vi "Resampler (2 Channel).vi"(5 "CalibrationTable Length-1":u16=799, 7 "ResampleVectorInfo":refnum<k21>="Interpolation Vector Table", 8 "DataValid":bool=TRUE, 11 "Input Data":T2[](array[typedef])=[0.0, 0.0]) -> (0 "Data Valid":bool[](array[boolean]), 3 "Interpolated Data":T1[](array[typedef]))   [LabVIEW 2011]
doc: "This VI resamples input stream to rquired input length of FFT.\n\nTable Length-1 is the length of calibration table. \nIf Input record length is 1600 and processing is done per 2 samples. Then Table-1 = 1600/2-1 = 799"
uses:
  <userlib>/FPGA Library/Code Development/Signal Processing/Interpolation Block/Controls/Interpolation Input Data.ctl
  <userlib>/FPGA Library/Code Development/Signal Processing/Interpolation Block/Controls/Interpolation Output Data.ctl
  <vilib>/rvi/DataTransferAndStorage/Container/Common/niFpgaContainerExecOnDevCompGetState.vi
  <vilib>/rvi/Memory/Memory_Emulation/niFpgaMemoryEmulationValidateCache.vi
  <vilib>/rvi/DataTransferAndStorage/Container/Common/niFpgaContainerGetUniqueNameForEmu.vi
  <vilib>/rvi/Memory/Memory_Emulation/nirvimemoryEmulationManagerCache_InsertValue.vi
  <vilib>/Utility/error.llb/Clear Errors.vi
  <vilib>/rvi/Memory/Memory_Emulation/nirvimemoryEmulationManagerCache_GetValue.vi
  <vilib>/rvi/FXPMathLib/basic elements/FxpDiscreteDelay/XNode/nifxpmath_DiscreteDelay.xnode
  <vilib>/rvi/DataTransferAndStorage/Container/XNode/niFpgaContainer.xnode
  <vilib>/rvi/Memory/Memory_Emulation/niFpgaMemoryEmulationRefIn.vi
  <userlib>/FPGA Library/Code Development/Signal Processing/Interpolation Block/Controls/ResampleVectorInfo (Single Point).ctl
  <userlib>/FPGA Library/Code Development/Signal Processing/Interpolation Block/Controls/ResampleVectorInfo (Multiple Point).ctl
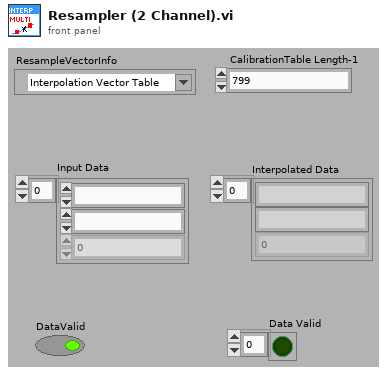
[diagram p1: front panel]
types:
  T1 = typedef "Interpolation Output Data.ctl" = fxp<+/-,19,1>
  T2 = typedef "Interpolation Input Data.ctl" = fxp<+/-,18,1>
  T3 = typedef "ResampleVectorInfo (Multiple Point).ctl" = cluster{"x[n].ResampleInfo":T4, "x[n-1].ResampleInfo":T4}
  T4 = typedef "ResampleVectorInfo (Single Point).ctl" = cluster{"Calc Resample?":bool, "Lambda":fxp<+/-,18,1>}
  T5 = cluster{"x[n].ResampleInfo":cluster{"Calc Resample?":bool, "Lambda":fxp<+/-,18,1>}, "x[n-1].ResampleInfo":cluster{"Calc Resample?":bool, "Lambda":fxp<+/-,18,1>}}
  T6 = cluster{"Calc Resample?":bool, "Lambda":fxp<+/-,18,1>}
  T7 = cluster{"Interpolated Value":T1, "Output Valid":bool}
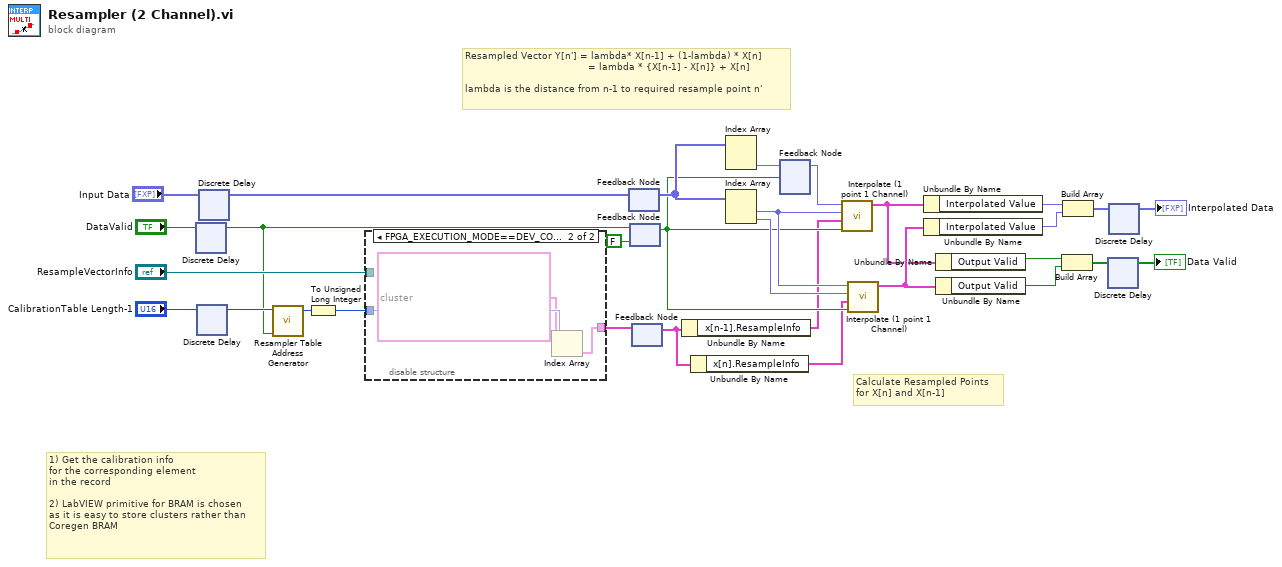
[diagram p0: block diagram]
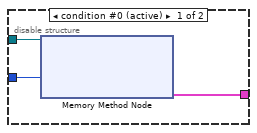
[diagram p2: hidden frame]
diagram:
  # "Calculate Resampled Points\nfor X[n] and X[n-1]"
  # "1) Get the calibration info\nfor the corresponding element\nin the record\n\n2) LabVIEW primitive for BRAM is chosen\nas it is easy to store clusters rather than\nCoregen BRAM"
  # "Resampled Vector Y[n'] = lambda* X[n-1] + (1-lambda) * X[n]\n                                         = lambda * {X[n-1] - X[n]} + X[n]\n\nlambda is the distance from n-1 to required resample point n'"
  n1 = xnode "Discrete Delay"("D"="DataValid") -> ("Q"=w5:bool)
  n2 = xnode "Discrete Delay"("D"="CalibrationTable Length-1") -> ("Q"=w6:u16)
  n3 = xnode "Discrete Delay"("D"="Input Data") -> ("Q"=w4:fxp<+/-,18,1>[])
  n4 = call <userlib>:"Resampler Table Address Generator.vi"("INC?"=w5, "Table Length"=w6) -> ("Read Address"=w26:u16)  [unwired: 9 in]
  n5 = To Unsigned Long Integer(number=w26) -> (unsigned 32bit integer=w25:u32)
  n6 = disable-structure shown="FPGA_EXECUTION_MODE==DEV_COMPUTER_SIM_IO, default" {
    disable-tunnel: "ResampleVectorInfo" -> [w33 _]
    disable-tunnel: [w32 w36] -> w29
    disable-tunnel: w25 -> [w31 w35]
    frame condition #0 (active) {
      n7 = xnode ("Memory Method Node")("Address"=w31, "Memory In"=w33) -> ("Data"=w32:T5)  [unwired: 1 out]
    }
    frame condition #1 {
      n8 = Index Array(array=T3[] data[14404B] ("Resample Vector Table"), index=w35) -> (element=w36:T3)
    }
  }
  n9 = feedback-in #1(w4) -> ()
  n10 = feedback #1() -> (w19:fxp<+/-,18,1>[])  [unwired: 1 in]
  n11 = feedback-in #2(w5) -> ()
  n12 = feedback #2(FALSE ("Q")) -> (w18:bool)
  n13 = feedback-in #3(w29) -> ()
  n14 = feedback #3() -> (w9:T5)  [unwired: 1 in]
  n15 = Unbundle By Name(w9) -> ("x[n-1].ResampleInfo"=w8:T6)
  n16 = Unbundle By Name(w9) -> ("x[n].ResampleInfo"=w7:T6)
  n17 = Index Array(array=w19) -> (element #2=w21:fxp<+/-,18,1>)  [unwired: 2 in, 1 out]
  n18 = Index Array(array=w19) -> (element #1=w24:fxp<+/-,18,1>, element #2=w23:fxp<+/-,18,1>)  [unwired: 2 in]
  n19 = feedback-in #4(w21, w18) -> ()
  n20 = feedback #4() -> (w20:fxp<+/-,18,1>)  [unwired: 1 in]
  n21 = call <userlib>:"Interpolate (1 point 1 Channel).vi"("Data Valid"=w18, "x[n].ResampleInfo"=w8, "Current Point.Value"=w24, "Previous Point.Value"=w20) -> ("Output Data"=w14:T7)  [unwired: 7 in]
  n22 = call <userlib>:"Interpolate (1 point 1 Channel).vi"("Data Valid"=w18, "x[n].ResampleInfo"=w7, "Current Point.Value"=w23, "Previous Point.Value"=w24) -> ("Output Data"=w15:T7)  [unwired: 7 in]
  n23 = Unbundle By Name(w14) -> ("Interpolated Value"=w17:T1)
  n24 = Unbundle By Name(w15) -> ("Interpolated Value"=w16:T1)
  n25 = Unbundle By Name(w14) -> ("Output Valid"=w13:bool)
  n26 = Unbundle By Name(w15) -> ("Output Valid"=w12:bool)
  n27 = Build Array(w13, w12) -> (w10:bool[])
  n28 = Build Array(w17, w16) -> (w11:T1[])
  n29 = xnode "Discrete Delay"("D"=w10) -> ("Q"=→"Data Valid":bool[])
  n30 = xnode "Discrete Delay"("D"=w11) -> ("Q"=→"Interpolated Data":fxp<+/-,19,1>[])
